vi "Set Stop Trigger (Analog Edge).vi"(7 "Post-Trigger Duration (0 s)":dbl, 8 "error in (no error)":errorcluster, 9 "Trigger Channel":string, 10 "Analog Edge Condition":T1, 11 "Data Logging Specification Ref in":T3) -> (0 "error out":errorcluster, 3 "Data Logging Specification Ref out":T3)   [LabVIEW 2020, in "NI_VS Data Logging API.lvlib"]
doc: "Specifies a trigger condition on which to stop logging data. You also can specify whether to continue logging channel data for a set period of time after the trigger condition occurs.\n\nYou must manually select the polymorphic instance to use."
uses:
  <vilib>/NI VeriStand/Execution/DataLogging/NI_VS Data Logging API.lvlib
  <vilib>/NI VeriStand/Execution/DataLogging/DataLoggingSpecification Ref.ctl
  NationalInstruments.VeriStand.ClientAPI
  <vilib>/NI VeriStand/Execution/DataLogging/Analog Edge Condition.ctl
  <vilib>/NI VeriStand/Execution/DataLogging/Slope.ctl
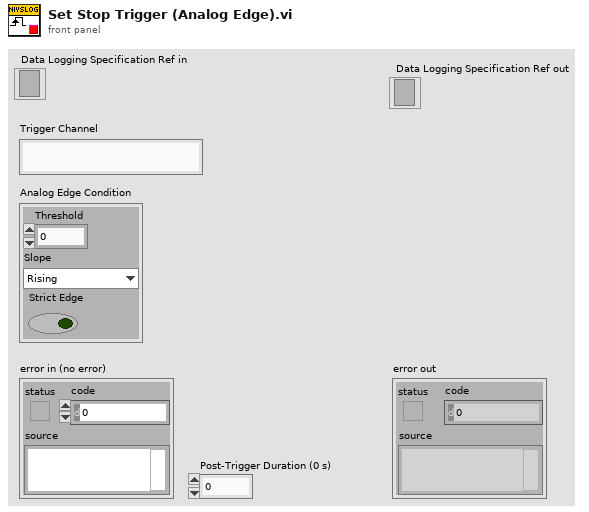
[diagram p1: front panel]
types:
  T1 = typedef "NI_VS Data Logging API.lvlib/Analog Edge Condition.ctl" = cluster{"Threshold":dbl, "Slope":T2, "Strict Edge":bool}
  T2 = typedef "NI_VS Data Logging API.lvlib/Slope.ctl" = enum16{"Rising", "Falling"}
  T3 = typedef "NI_VS Data Logging API.lvlib/DataLoggingSpecification Ref.ctl" = refnum<k24>
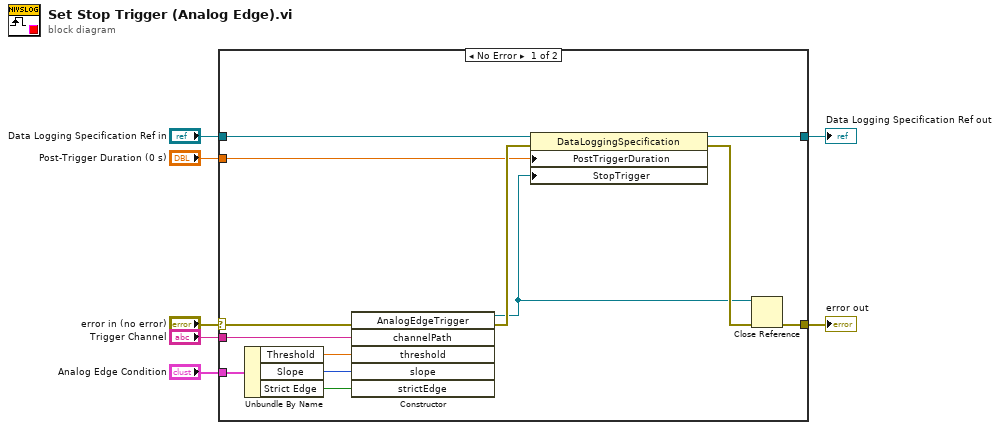
[diagram p0: block diagram]
diagram:
  n1 = case shown="No Error" "error in (no error)" {
    selector: "error in (no error)" -> [w17 w22]
    tunnel: "Trigger Channel" -> [w16 _]
    tunnel: "Data Logging Specification Ref in" -> [w18 w21]
    tunnel: [w9 w21] -> w5
    tunnel: [w8 w22] -> w4
    tunnel: "Post-Trigger Duration (0 s)" -> [w10 _]
    tunnel: "Analog Edge Condition" -> [w14 _]
    frame No Error {
      n2 = Unbundle By Name(w14) -> ("Threshold"=w13:dbl, "Slope"=w12:T2, "Strict Edge"=w11:bool)
      n3 = constructor class="AnalogEdgeTrigger"(error in=w17, "channelPath"=w16, "threshold"=w13, "slope"=w12, "strictEdge"=w11) -> (reference out=w15:refnum<k24>, error out=w20:errorcluster)  [unwired: 2 in, 5 out]
      n4 = property class="DataLoggingSpecification"(reference=w18, error in=w20, "PostTriggerDuration"=w10, "StopTrigger"=w15) -> (reference out=w9:T3, error out=w19:errorcluster)
      n5 = Close Reference(reference=w15, error in (no error)=w19) -> (error out=w8:errorcluster)
    }
    frame Error {
    }
  }
  "error out" <- w4
  "Data Logging Specification Ref out" <- w5
